vi "Key Control.vi"(8 "error in (no error)":errorcluster, 11 "Key Up? (F)":bool) -> (0 "error out":errorcluster, 3 "Up/Down":u32)   [LabVIEW 2020, in "MacroAssert.lvlib" / "Win Util.lvlib"]
uses:
  Win Util.lvlib
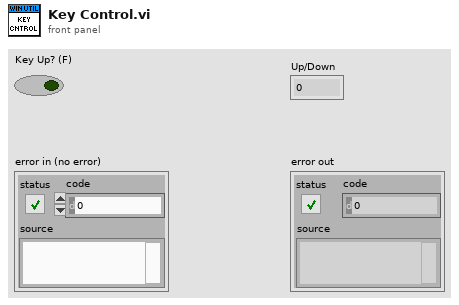
[diagram p1: front panel]
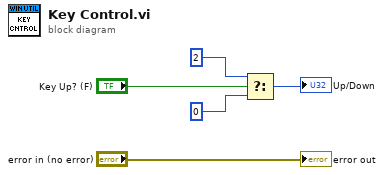
[diagram p0: block diagram]
diagram:
  n1 = Select(t=u32 2 ("Flags"), s="Key Up? (F)", f=u32 0 ("Flags")) -> (s? t:f=→"Up/Down":u32)
  "error out" <- "error in (no error)"
